vi "Cleanup Session.vi"(8 "error in":errorcluster, 11 "Plugin in":refnum<class "StreamReader.lvclass">) -> (0 "error out":errorcluster, 3 "Plugin out":refnum<class "StreamReader.lvclass">)   [LabVIEW 2024, in "StreamReader.lvlib" / "StreamReader.lvclass"]
uses:
  StreamReader.lvclass
  StreamReader.lvclass/StreamReader.ctl
  StreamReader Strings.vi
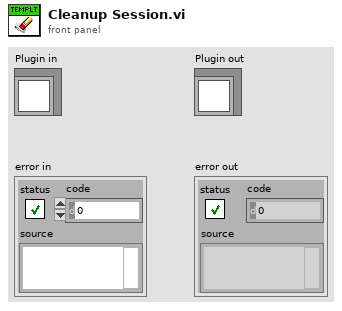
[diagram p1: front panel]
types:
  T1 = typedef "StreamReader.lvlib/StreamReader.lvclass/StreamReader Parameters.ctl" = cluster{"Reader URL":string, "Writer URL":string, "Buffer Size":i32, "Reader endpoint":refnum<k21>, "Channel Names":string[]}
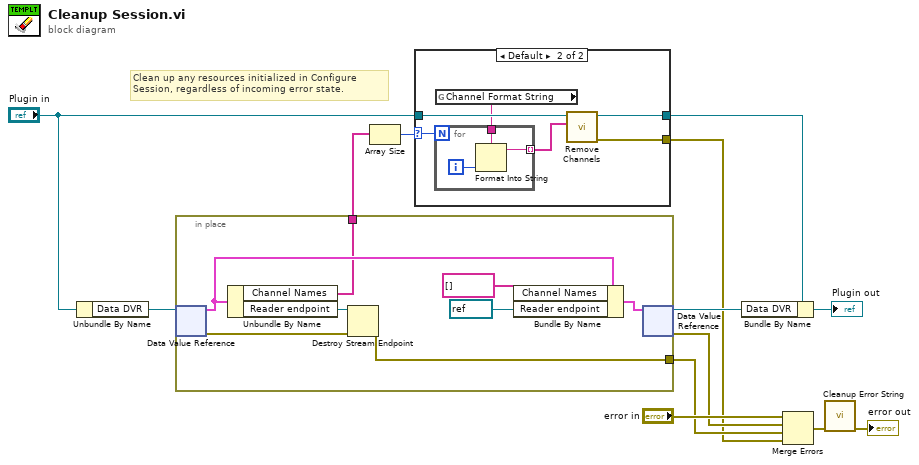
[diagram p0: block diagram]
diagram:
  # "Clean up any resources initialized in Configure Session, regardless of incoming error state."
  n1 = Unbundle By Name("Plugin in") -> ("Data DVR"=w12:refnum<data-value>)
  n2 = in-place {
    in-place-border: [w16] -> w8
    in-place-border: [w14] -> w6
    n3 = in-place-dvr #1(w12) -> (w19:T1, w20:errorcluster)
    n4 = Unbundle By Name(w19) -> ("Channel Names"=w14:string[], "Reader endpoint"=w21:refnum<k21>)
    n5 = Destroy Stream Endpoint(8:w20, 11:w21) -> (0:w16:errorcluster)
    n6 = Bundle By Name(cluster=w19, "Channel Names"=string[] [], "Reader endpoint"=refnum<k21> refnum) -> (w17:T1)
    n7 = in-place-dvr #1(w17) -> (w11:refnum<data-value>, w9:errorcluster)
  }
  n8 = Array Size(array=w6) -> (size(s)=w3:i32)
  n9 = case shown="Default" w3 {
    selector: w3 -> [_ w24]
    tunnel: "Plugin in" -> [w22 w27]
    tunnel: [_ w26] -> w4
    tunnel: [w22 w25] -> w5
    frame 0 {
    }
    frame Default {
      n10 = global read "StreamReader Strings.vi" "Channel Format String"() -> (w23:string)
      n11 = for {
        N: w24 -> [_]
        tunnel: [w31] -> w28 mode=indexing
        tunnel: w23 -> [w29]
        i -> [w30]
        n12 = Format Into String(format string=w29, w30) -> (resulting string=w31:string)  [unwired: 2 in, 1 out]
      }
      n13 = call-dynamic "Remove Channels.vi"("Unique Channel Identifiers to Delete"=w28, "Plugin in"=w27) -> ("error out"=w26:errorcluster, "Plugin out"=w25:refnum<class "StreamReader.lvclass">)  [unwired: 8 in]
    }
  }
  n14 = Bundle By Name(cluster=w5, "Data DVR"=w11) -> (→"Plugin out":refnum<class "StreamReader.lvclass">)
  n15 = Merge Errors("error in", w9, w8, w4) -> (w2:errorcluster)
  n16 = call "Cleanup Error String.vi"("error in (no error)"=w2) -> ("error out"=→"error out":errorcluster)  [unwired: 10 in]
